vi "nanostage-main.vi"() -> ()   [LabVIEW 2015]
panel:
  in  "switch L/R":bool
  in  "switch U/D":bool
  in  "xy stepsize":dbl=2.0 format="%.3f"
  in  "z-stepsize":dbl=0.25 format="%.3f"
  out "error message":string
  out "error":bool=TRUE
  in  "stop":bool
  out "plot x/y-position":cluster{dbl, dbl}[](graph)
  in  "z-axis":dbl=150.0 min=0.0 max=300.0 step=0.25 format="%.3f"
  in  "y-axis":dbl=150.0 min=0.0 max=300.0 step=2.0 format="%.3f"
  in  "x-axis":dbl=150.0 min=0.0 max=300.0 step=2.0 format="%.3f"
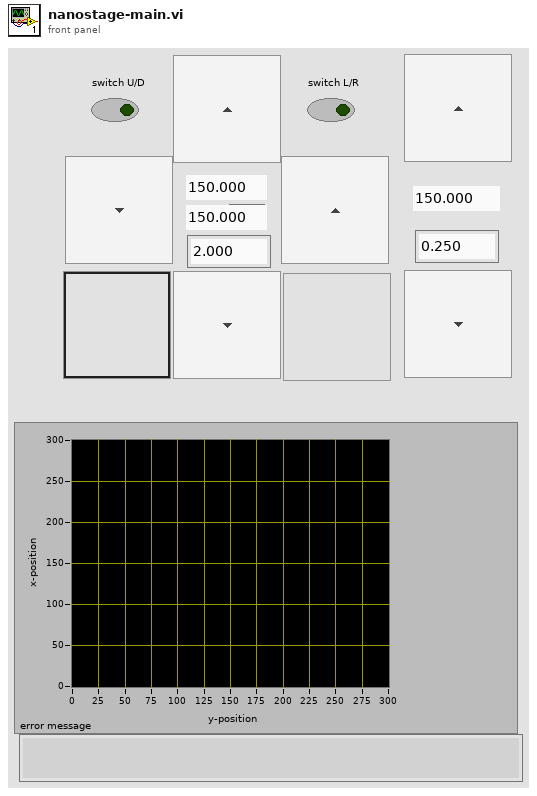
[diagram p1: front panel]
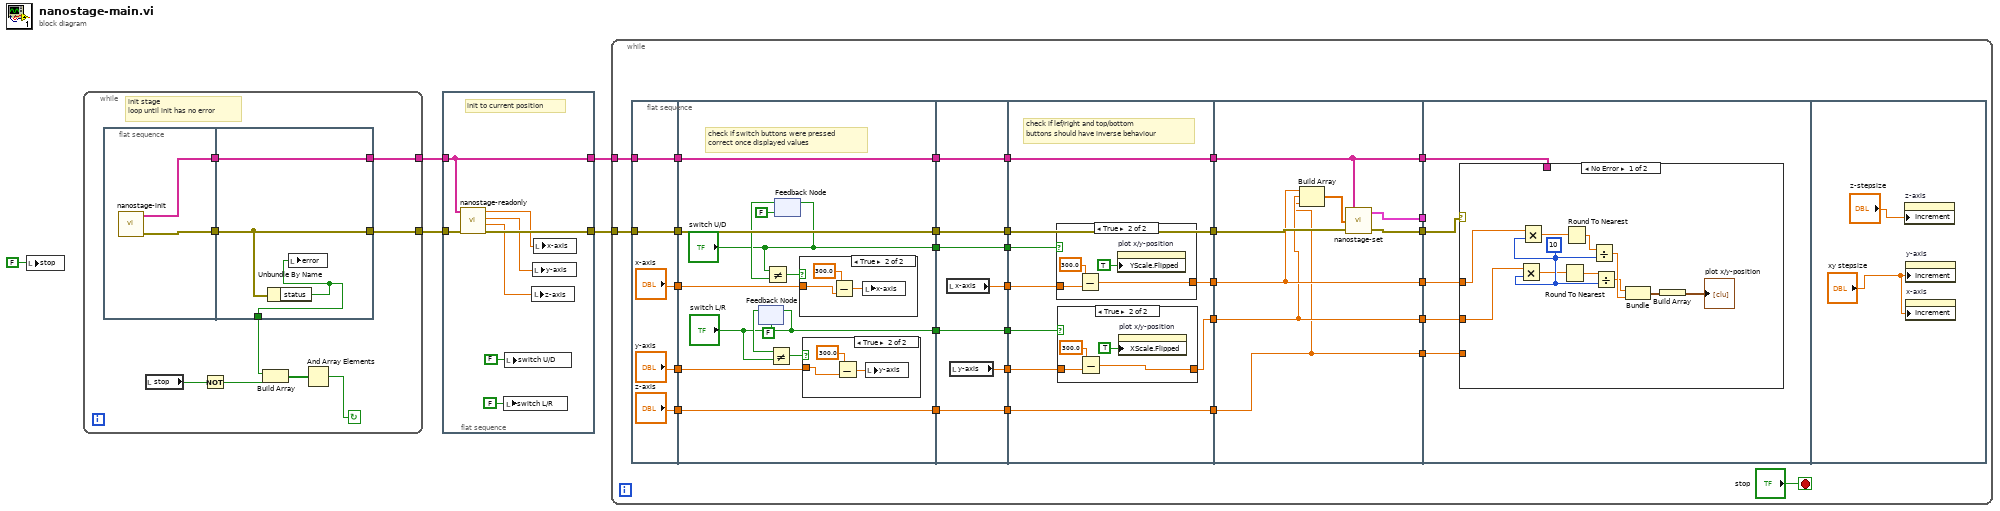
[diagram p0: block diagram]
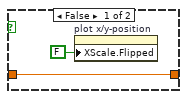
[diagram p4: hidden frame]
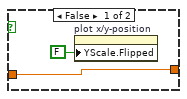
[diagram p5: hidden frame]
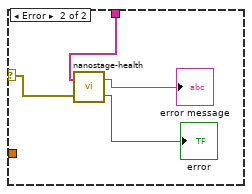
[diagram p6: hidden frame]
diagram:
  n1 = local write "stop"(FALSE ("stop")) -> ()
  n2 = while {
    tunnel: [w14] -> w4
    tunnel: [w13] -> w2
    stop <- w8 continue-if-true
    # "init stage\nloop until init has no error"
    n3 = flat-sequence {
      tunnel: [w16] -> w12
      tunnel: [w15] -> w11
      tunnel: [w19] -> w13
      tunnel: [w18] -> w14
      tunnel: w12 -> [w18]
      tunnel: w11 -> [w19]
      tunnel: [w17] -> w6
      frame #0 {
        n4 = call "nanostage-init.vi"() -> ("error out"=w16:errorcluster, "All conn. axes"=w15:string[])  [unwired: 4 in]
      }
      frame #1 {
        n5 = Unbundle By Name(w18) -> ("status"=w17:bool)
        n6 = local write "error"(w17) -> ()
      }
    }
    n7 = local read "stop"() -> (w7:bool)
    n8 = Not(x=w7) -> (.not. x?=w10:bool)
    n9 = Build Array(w6, w10) -> (w9:bool[])
    n10 = And Array Elements(Boolean array=w9) -> (logical AND=w8:bool)
  }
  n11 = flat-sequence {
    tunnel: w4 -> [w27]
    tunnel: [w26] -> w3
    tunnel: w2 -> [w25]
    tunnel: [w25] -> w1
    frame #0 {
      # "init to current position"
      n12 = call "nanostage-readonly.vi"("error in"=w27, "Axes to move"=w25) -> ("error out"=w26:errorcluster, "position-z"=w22:dbl, "position-y"=w23:dbl, "position-x"=w24:dbl)  [unwired: 2 in]
      n13 = local write "switch L/R"(FALSE ("switch L/R")) -> ()
      n14 = local write "switch U/D"(FALSE ("switch U/D")) -> ()
      n15 = local write "z-axis"(w22) -> ()
      n16 = local write "y-axis"(w23) -> ()
      n17 = local write "x-axis"(w24) -> ()
    }
  }
  n18 = while {
    tunnel: w3 -> [w58]
    tunnel: w1 -> [w51]
    stop <- "stop" stop-if-true
    n19 = flat-sequence {
      tunnel: w51 -> [w62]
      tunnel: w58 -> [w63]
      tunnel: [w63] -> w44
      tunnel: [w62] -> w43
      tunnel: ["x-axis"] -> w42
      tunnel: ["y-axis"] -> w41
      tunnel: ["z-axis"] -> w40
      tunnel: [w76] -> w39
      tunnel: [w75] -> w37
      tunnel: [w74] -> w33
      tunnel: w44 -> [w76]
      tunnel: w43 -> [w75]
      tunnel: w42 -> [w69]
      tunnel: w41 -> [w64]
      tunnel: w40 -> [w74]
      tunnel: ["switch U/D"] -> w31
      tunnel: ["switch L/R"] -> w29
      tunnel: w39 -> [w89]
      tunnel: [w89] -> w38
      tunnel: w37 -> [w88]
      tunnel: [w88] -> w36
      tunnel: [w84] -> w35
      tunnel: [w83] -> w34
      tunnel: w33 -> [w87]
      tunnel: [w87] -> w32
      tunnel: w31 -> [w86]
      tunnel: [w86] -> w30
      tunnel: w29 -> [w85]
      tunnel: [w85] -> w28
      tunnel: w38 -> [w98]
      tunnel: [w98] -> w49
      tunnel: w36 -> [w97]
      tunnel: [w97] -> w48
      tunnel: w35 -> [w90]
      tunnel: [w96] -> w47
      tunnel: w34 -> [w95]
      tunnel: [w94] -> w46
      tunnel: w32 -> [w94]
      tunnel: [w93] -> w45
      tunnel: w30 -> [w92]
      tunnel: w28 -> [w91]
      tunnel: [w116] -> w57
      tunnel: [w118] -> w56
      tunnel: [w117] -> w55
      tunnel: [w112] -> w54
      tunnel: [w113] -> w53
      tunnel: [w114] -> w52
      tunnel: w49 -> [w115]
      tunnel: w48 -> [w117]
      tunnel: w47 -> [w114]
      tunnel: w46 -> [w112]
      tunnel: w45 -> [w113]
      tunnel: w57 -> [_]
      tunnel: w56 -> [w119]
      tunnel: w55 -> [w123]
      tunnel: w54 -> [w122]
      tunnel: w53 -> [w121]
      tunnel: w52 -> [w120]
      frame #0 {
      }
      frame #1 {
        # "check if switch buttons were pressed\ncorrect once displayed values"
        n20 = feedback #1(FALSE ("switch U/D")) -> (w67:bool)
        n21 = feedback-in #1("switch L/R") -> ()
        n22 = Not Equal?(x=w67, y="switch L/R") -> (x != y?=w65:bool)
        n23 = feedback-in #2("switch U/D") -> ()
        n24 = feedback #2(FALSE ("switch U/D")) -> (w72:bool)
        n25 = Not Equal?(x="switch U/D", y=w72) -> (x != y?=w70:bool)
        n26 = case shown="True" w70 {
          tunnel: w69 -> [_ w82]
          frame False {
          }
          frame True {
            n27 = Subtract(x=300.0, y=w82) -> (x-y=w80:dbl)
            n28 = local write "x-axis"(w80) -> ()
          }
        }
        n29 = case shown="True" w65 {
          tunnel: w64 -> [_ w77]
          frame False {
          }
          frame True {
            n30 = Subtract(x=300.0, y=w77) -> (x-y=w78:dbl)
            n31 = local write "y-axis"(w78) -> ()
          }
        }
      }
      frame #2 {
        n32 = local read "x-axis"() -> (w84:dbl)
        n33 = local read "y-axis"() -> (w83:dbl)
      }
      frame #3 {
        # "check if lef/right and top/bottom\nbuttons should have inverse behaviour"
        n34 = case shown="True" w92 {
          tunnel: w90 -> [w106 w109]
          tunnel: [w106 w108] -> w96
          frame False {
            n35 = property on="plot x/y-position" class="XYGraph (strict)"("YScale.Flipped"=FALSE ("Y Scale.Flipped")) -> ()  [unwired: 2 in, 2 out]
          }
          frame True {
            n36 = Subtract(x=300.0, y=w109) -> (x-y=w108:dbl)
            n37 = property on="plot x/y-position" class="XYGraph (strict)"("YScale.Flipped"=TRUE ("Y Scale.Flipped")) -> ()  [unwired: 2 in, 2 out]
          }
        }
        n38 = case shown="True" w91 {
          tunnel: w95 -> [w100 w103]
          tunnel: [w100 w102] -> w93
          frame False {
            n39 = property on="plot x/y-position" class="XYGraph (strict)"("XScale.Flipped"=FALSE ("Y Scale.Flipped")) -> ()  [unwired: 2 in, 2 out]
          }
          frame True {
            n40 = Subtract(x=300.0, y=w103) -> (x-y=w102:dbl)
            n41 = property on="plot x/y-position" class="XYGraph (strict)"("XScale.Flipped"=TRUE ("Y Scale.Flipped")) -> ()  [unwired: 2 in, 2 out]
          }
        }
      }
      frame #4 {
        n42 = Build Array(w114, w113, w112) -> (w111:dbl[])
        n43 = call "nanostage-set.vi"("error in"=w115, "setValues"=w111, "Axes to move"=w117) -> ("error out"=w118:errorcluster, "getValues"=w116:cluster{"postion":dbl[], "status":bool[]})  [unwired: 1 out]
      }
      frame #5 {
        n44 = case shown="No Error" w119 {
          selector: w119 -> [_ w138]
          tunnel: w123 -> [_ w137]
          tunnel: w122 -> [_ _]
          tunnel: w121 -> [w124 _]
          tunnel: w120 -> [w125 _]
          frame No Error {
            w132 = 10
            n45 = Multiply(x=w124, y=w132) -> (x*y=w131:dbl)
            n46 = Multiply(x=w125, y=w132) -> (x*y=w128:dbl)
            n47 = Round To Nearest(number=w131) -> (nearest integer value=w130:dbl)
            n48 = Round To Nearest(number=w128) -> (nearest integer value=w129:dbl)
            n49 = Divide(x=w129, y=w132) -> (x/y=w134:dbl)
            n50 = Divide(x=w130, y=w132) -> (x/y=w133:dbl)
            n51 = Bundle(w133, w134) -> (w127:cluster{dbl, dbl})  [unwired: 1 in]
            n52 = Build Array(w127) -> (→"plot x/y-position":cluster{dbl, dbl}[])
          }
          frame Error {
            n53 = call "nanostage-health.vi"("error in"=w138, "All conn. axes"=w137) -> ("error"=→"error":bool, "error message"=→"error message":string)
          }
        }
      }
      frame #6 {
        n54 = property on="z-axis" class="DigNum (strict)"("Increment"="z-stepsize") -> ()  [unwired: 2 in, 2 out]
        n55 = property on="y-axis" class="DigNum (strict)"("Increment"="xy stepsize") -> ()  [unwired: 2 in, 2 out]
        n56 = property on="x-axis" class="DigNum (strict)"("Increment"="xy stepsize") -> ()  [unwired: 2 in, 2 out]
      }
    }
  }
